vi "Do Rename Object.vi"(8 "error in (no error)":errorcluster, 10 "rename_object Argument":T2, 11 "Data Cluster in":T1) -> (0 "error out":errorcluster, 3 "Data Cluster out":T1)   [LabVIEW 2025, in "Scripting Server.lvlib"]
uses:
  Scripting Server.lvlib
  rename_object Argument--cluster.ctl
  rename_object (Reply Payload)--cluster.ctl
  Module Data--cluster.ctl
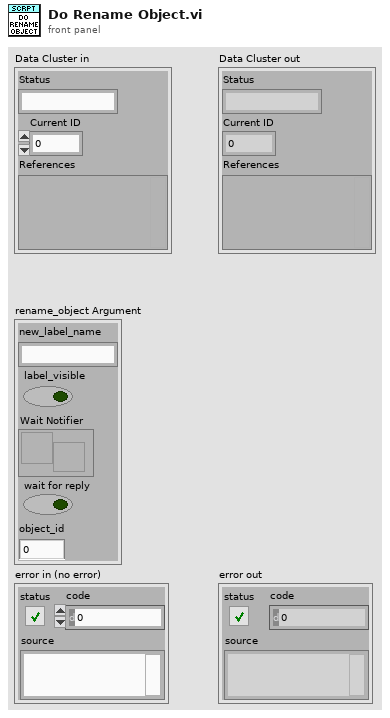
[diagram p1: front panel]
types:
  T1 = typedef "Scripting Server.lvlib/Module Data--cluster.ctl" = cluster{"Status":string, "Current ID":i32, "References":variant}
  T2 = typedef "Scripting Server.lvlib/rename_object Argument--cluster.ctl" = cluster{"new_label_name":string, "label_visible":bool, "Wait Notifier":refnum<notifier>, "wait for reply":bool, "object_id":i32}
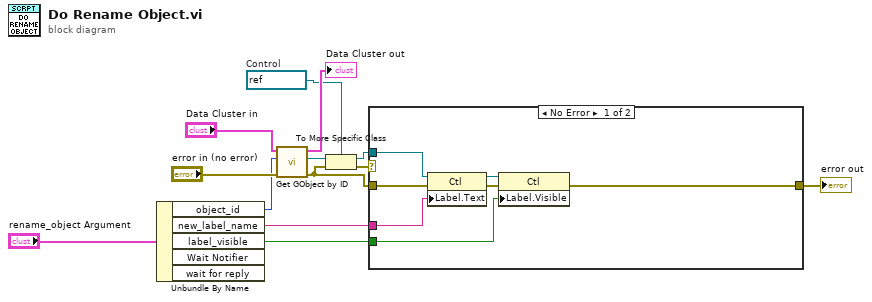
[diagram p0: block diagram]
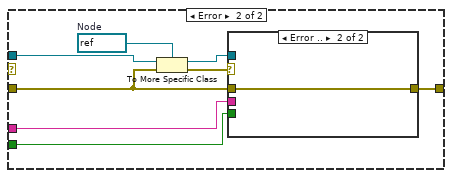
[diagram p2: hidden frame]
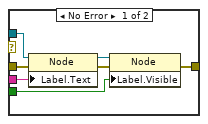
[diagram p3: hidden frame]
diagram:
  w6 = refnum<vi> refnum  # Control
  n1 = Unbundle By Name("rename_object Argument") -> ("object_id"=w9:i32, "new_label_name"=w5:string, "label_visible"=w3:bool)  [unwired: 2 out]
  n2 = call "Get GObject by ID.vi"("error in (no error)"="error in (no error)", "ID"=w9, "Data Cluster in"="Data Cluster in") -> ("error out"=w1:errorcluster, "gobject"=w8:refnum<vi>, "Data Cluster out"=→"Data Cluster out":T1)  [unwired: 6 in]
  n3 = To More Specific Class(target class=w6, reference=w8, error in=w1) -> (specific class reference=w7:refnum<vi>, error out=w4:errorcluster)
  n4 = case shown="No Error" w4 {
    tunnel: w7 -> [w20 w28]
    tunnel: w5 -> [w19 w22]
    tunnel: w3 -> [w17 w23]
    tunnel: [w16 w26] -> w2
    tunnel: w1 -> [w14 w21]
    frame No Error {
      n5 = property class="Ctl"(reference=w20, error in=w14, "Label.Text"=w19) -> (reference out=w18:refnum<vi>, error out=w15:errorcluster)
      n6 = property class="Ctl"(reference=w18, error in=w15, "Label.Visible"=w17) -> (error out=w16:errorcluster)  [unwired: 1 out]
    }
    frame Error {
      w27 = refnum<vi> refnum  # Node
      n7 = To More Specific Class(target class=w27, reference=w28, error in=w21) -> (specific class reference=w24:refnum<vi>, error out=w25:errorcluster)
      n8 = case shown="Error .." w25 {
        tunnel: [w33 w36] -> w26
        tunnel: w24 -> [w34 _]
        tunnel: w23 -> [w31 _]
        tunnel: w22 -> [w30 _]
        tunnel: w21 -> [w29 w36]
        frame No Error {
          n9 = property class="Node"(reference=w34, error in=w29, "Label.Text"=w30) -> (reference out=w32:refnum<vi>, error out=w35:errorcluster)
          n10 = property class="Node"(reference=w32, error in=w35, "Label.Visible"=w31) -> (error out=w33:errorcluster)  [unwired: 1 out]
        }
        frame Error {
        }
      }
    }
  }
  "error out" <- w2
